vi "Bulk Add AO Register - Right Click.vi"(11 "Node Ptr":T1 format="%.0x") -> ()   [LabVIEW 2015, in "Modbus Master System Explorer.lvlib"]
uses:
  Modbus Master System Explorer.lvlib
  <vilib>/NI Veristand/Custom Device API/Custom Device Item Ref.ctl
  SubVIs/Modbus Type.ctl
  Shared/Controls/Data Model/Mapping.ctl
  Shared/Controls/Data Model/DataType.ctl
  Shared/Modbus Master Shared.lvlib
  <vilib>/NI VeriStand/Custom Device API/Custom Device API.lvlib
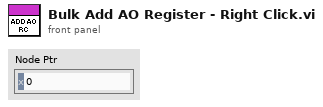
[diagram p1: front panel]
types:
  T1 = typedef "Custom Device API.lvlib/Custom Device Item Ref.ctl" = u64
  T2 = typedef "Modbus Master Shared.lvlib/Modbus Type.ctl" = enum16{"Coil", "Discrete Input", "Holding Register", "Input Register"}
  T3 = typedef "Modbus Master Shared.lvlib/DataType.ctl" = enum16{"Double", "Single", "I64", "I32", "I16", "I8", "U64", "U32", "U16", "U8", "Boolean"}
  T4 = typedef "Modbus Master Shared.lvlib/Mapping.ctl" = cluster{"DataType":T3, "Starting Address":u16, "Sub-Index (Bool)":u16, "VS Reference":T1}
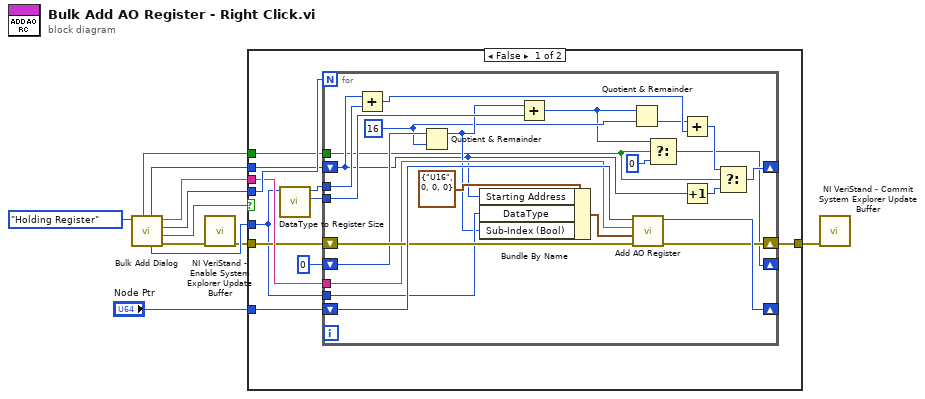
[diagram p0: block diagram]
diagram:
  n1 = call "Bulk Add Dialog.vi"("Type"=Modbus_Type."Holding Register") -> ("error out"=w4:errorcluster, "Cancelled?"=w8:bool, "Quantity Out"=w9:u16, "Root Name Out"=w10:string, "DataType Out"=w7:T3, "Starting Address Out"=w11:u16, "Pack Values? Out"=w5:bool)  [unwired: 4 in]
  n2 = call <vilib>:"NI VeriStand - Enable System Explorer Update Buffer.vi"("error in (no error)"=w4) -> ("error out"=w3:errorcluster)  [unwired: 10 in]
  n3 = case shown="False" w8 {
    tunnel: "Node Ptr" -> [w15 _]
    tunnel: w9 -> [w22 _]
    tunnel: w3 -> [w16 w46]
    tunnel: w10 -> [w21 _]
    tunnel: w11 -> [w20 _]
    tunnel: w7 -> [w14 _]
    tunnel: w5 -> [w13 _]
    tunnel: [w12 w46] -> w2
    frame False {
      n4 = call "DataType to Register Size.vi"("DataType"=w14) -> ("bits"=w17:i32, "bytes"=w19:i32)  [unwired: 9 in]
      n5 = for {
        N: w22 -> [_]
        shift-right: [w43] -> _
        shift-left: w15 -> [w45]
        shift-right: [w41] -> w12
        shift-left: w16 -> [w44]
        tunnel: w21 -> [w42]
        shift-right: [w28] -> _
        shift-left: w20 -> [w30]
        tunnel: w14 -> [w39]
        tunnel: w19 -> [w38]
        shift-right: [w25] -> _
        shift-left: 0 ("Sub-Index (Bool)") -> [w36]
        tunnel: w17 -> [w37]
        tunnel: w13 -> [w27]
        w33 = 16 ("y")
        n6 = Add(x=w30, y=w38) -> (x+y=w34:i32)
        n7 = Quotient & Remainder(x=w36, y=w33) -> (x-y*floor(x/y)=w35:i32)  [unwired: 1 out]
        n8 = Bundle By Name(cluster=T4 {"DataType"=enum."U16", "Starting Address"=0, "Sub-Index (Bool)"=0, "VS Reference"=0} ("Mapping"), "Starting Address"=w30, "DataType"=w39, "Sub-Index (Bool)"=w35) -> (w23:T4)
        n9 = Add(x=w35, y=w37) -> (x+y=w26:i32)
        n10 = Quotient & Remainder(x=w26, y=w33) -> (floor(x/y)=w32:i32)  [unwired: 1 out]
        n11 = call "Add AO Register.vi"("error in (no error)"=w44, "Mapping"=w23, "Label"=w42, "Node Ref In"=w45) -> ("error out"=w41:errorcluster, "Node Ref out"=w43:T1)  [unwired: 5 in, 1 out]
        n12 = Select(t=w26, s=w27, f=0 ("t")) -> (s? t:f=w25:i32)
        n13 = Add(x=w32, y=w34) -> (x+y=w29:i32)
        n14 = Increment(x=w30) -> (x+1=w31:i32)
        n15 = Select(t=w29, s=w27, f=w31) -> (s? t:f=w28:i32)
      }
    }
    frame True {
    }
  }
  n16 = call <vilib>:"NI VeriStand - Commit System Explorer Update Buffer.vi"("error in (no error)"=w2) -> ()  [unwired: 10 in, 1 out]
